vi "Create_sine_cosine.vi"(10 "Frequency":dbl, 11 "Waveform Data":waveform(dbl)) -> (2 "Array 2":dbl[](array[numeric]), 3 "Array":dbl[](array[numeric]))   [LabVIEW 2015]
uses:
  <vilib>/Waveform/WDTOps.llb/WDT Get Waveform Time Array DBL.vi
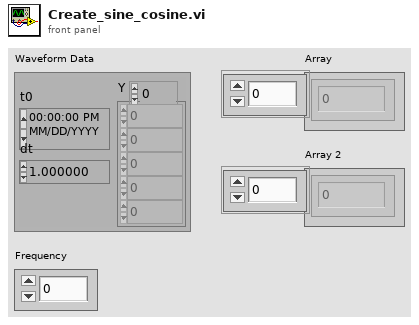
[diagram p1: front panel]
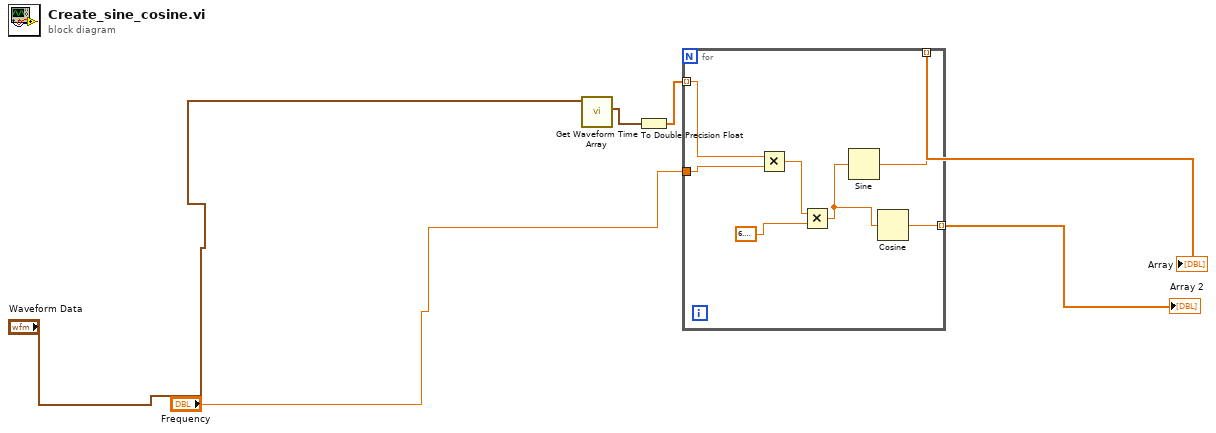
[diagram p0: block diagram]
diagram:
  n1 = call-poly <vilib>:"Get Waveform Time Array.vi"("waveform in"="Waveform Data") -> ("X array"=w2:timestamp[])  [unwired: 9 in, 1 out]
  n2 = To Double Precision Float(number=w2) -> (double precision float=w3:dbl[])
  n3 = for {
    tunnel: w3 -> [w13] mode=indexing
    tunnel: "Frequency" -> [w12]
    tunnel: [w11] -> w6 mode=indexing
    tunnel: [w7] -> w5 mode=indexing
    n4 = Multiply(x=w13, y=w12) -> (x*y=w9:dbl)
    n5 = Multiply(x=w9, y=6.283185307179586) -> (x*y=w8:dbl)
    n6 = Sine(x=w8) -> (sin(x)=w11:dbl)
    n7 = Cosine(x=w8) -> (cos(x)=w7:dbl)
  }
  "Array" <- w6
  "Array 2" <- w5
